vi "Create OS Specific Parameters.vi"(8 "error in (no error)":errorcluster, 11 "Compiled.Settings":T1={"Name"="", "Decimation"=0, "Channel Names"=[], "Hosted IP Address"="", "Hosted Port"=8382, "gRPC Port"=53251}) -> (0 "error out":errorcluster, 1 "json path":path, 2 "webpage directory":path, 3 "start cmd":string, 5 "gRPC address":string)   [LabVIEW 2026, in "WebPage Addon Engine.lvlib"]
uses:
  WebPage Addon Engine.lvlib
  Addon Shared/Types/Compiled.Settings.ctl
  Addon Shared/WebPage Addon Shared.lvlib
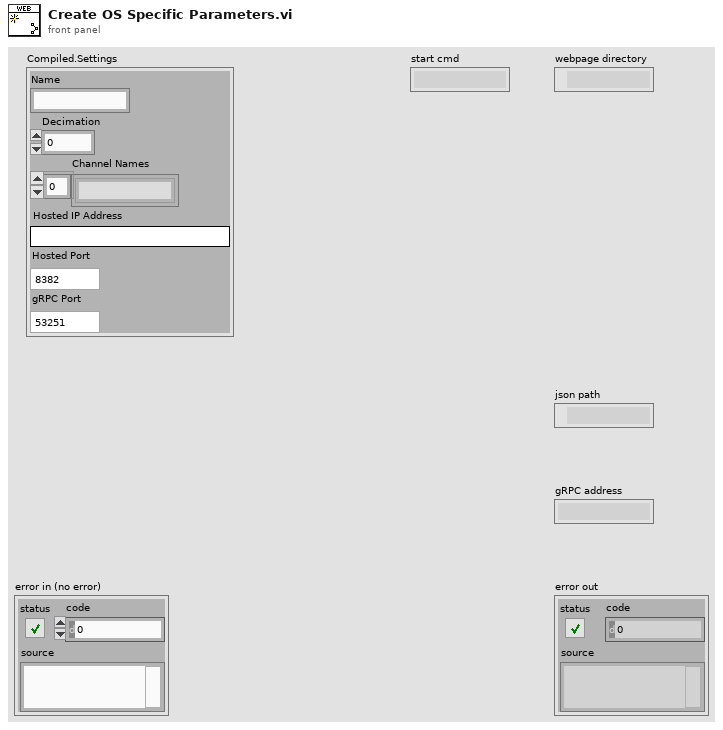
[diagram p1: front panel]
types:
  T1 = typedef "WebPage Addon Shared.lvlib/Compiled.Settings.ctl" = cluster{"Name":string, "Decimation":u32, "Channel Names":string[], "Hosted IP Address":string, "Hosted Port":u32, "gRPC Port":u32}
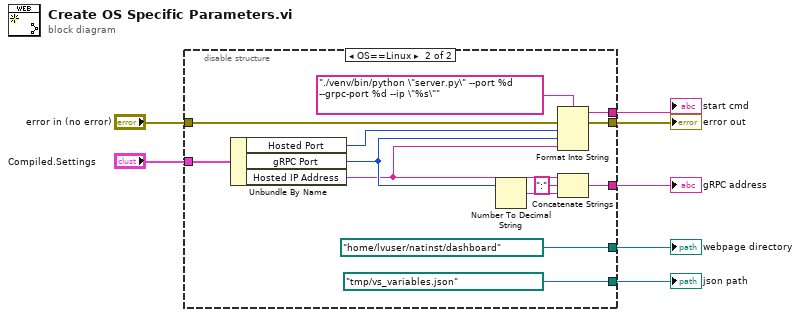
[diagram p0: block diagram]
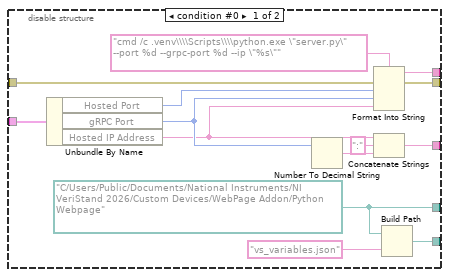
[diagram p2: hidden frame]
diagram:
  n1 = disable-structure shown="OS==Linux" {
    disable-tunnel: [w17 w23] -> w5
    disable-tunnel: [w21 path "/home/lvuser/natinst/dashboard" ("working directory")] -> w7
    disable-tunnel: [w20 path "/tmp/vs_variables.json" ("path")] -> w1
    disable-tunnel: "Compiled.Settings" -> [w16 w26]
    disable-tunnel: [w10 w22] -> w6
    disable-tunnel: "error in (no error)" -> [w9 w27]
    disable-tunnel: [w8 w25] -> w4
    frame condition #0 {
      w21 = path "C:/Users/Public/Documents/National Instruments/NI VeriStand 2026/Custom Devices/WebPage Addon/Python Webpage" ("working directory")
      n2 = Unbundle By Name(w16) -> ("Hosted Port"=w15:u32, "gRPC Port"=w14:u32, "Hosted IP Address"=w13:string)
      n3 = Number To Decimal String(number=w14) -> (decimal integer string=w12:string)  [unwired: 1 in]
      n4 = Format Into String(format string="cmd /c .venv\\\\Scripts\\\\python.exe \"server.py\" --port %d --grpc-port %d --ip \"%s\"" ("command line"), error in=w9, w15, w14, w13) -> (resulting string=w17:string, error out=w8:errorcluster)  [unwired: 1 in]
      n5 = Concatenate Strings(w13, ":" ("string"), w12) -> (w10:string)
      n6 = Build Path(base path=w21, name or relative path="vs_variables.json" ("command line")) -> (appended path=w20:path)
    }
    frame condition #1 (active) {
      n7 = Unbundle By Name(w26) -> ("Hosted Port"=w32:u32, "gRPC Port"=w31:u32, "Hosted IP Address"=w30:string)
      n8 = Number To Decimal String(number=w31) -> (decimal integer string=w29:string)  [unwired: 1 in]
      n9 = Format Into String(format string="./venv/bin/python \"server.py\" --port %d --grpc-port %d --ip \"%s\"" ("command line"), error in=w27, w32, w31, w30) -> (resulting string=w23:string, error out=w25:errorcluster)  [unwired: 1 in]
      n10 = Concatenate Strings(w30, ":" ("string"), w29) -> (w22:string)
    }
  }
  "webpage directory" <- w7
  "gRPC address" <- w6
  "start cmd" <- w5
  "error out" <- w4
  "json path" <- w1
